vi "GetCutData.vi"(8 "error in (no error)":errorcluster, 9 "CustomMarking":T1={"CustomMarkVar"="JointAngles", "CustomMarkVarIdx"=0}, 10 "CutVar":T2, 11 "CAlexData":refnum<class "CAlex2_Data.lvclass">) -> (0 "error out":errorcluster, 1 "MarkingVar":dbl[](array[numeric]), 2 "Time":dbl[](array[numeric]), 3 "CAlexData out":refnum<class "CAlex2_Data.lvclass">, 4 "MarkingVar3":dbl[][](array[numeric]))   [LabVIEW 2016, in "CAlex2_Data.lvclass"]
uses:
  CAlex2_Data.lvclass
  cutvar.ctl
  D:/JinXin/LabVIEW.git/CAlex2-Controller-master/Sim&Process/DataProcess/ExpData/ExpData.lvclass
  CAlex2_Data.lvclass/CAlex2_Data.ctl
  Classes/CAlex2/CAlex2.lvclass
  D:/JinXin/LabVIEW.git/CAlex2-Controller-master/Classes/SerialChain-Cable/SerialChain-Cable.lvclass
  ExpData/ExpData.lvclass
  Classes/SerialChain-Cable/SerialChain-Cable.lvclass
panel:
  out "Waveform Graph":dbl[][](graph)
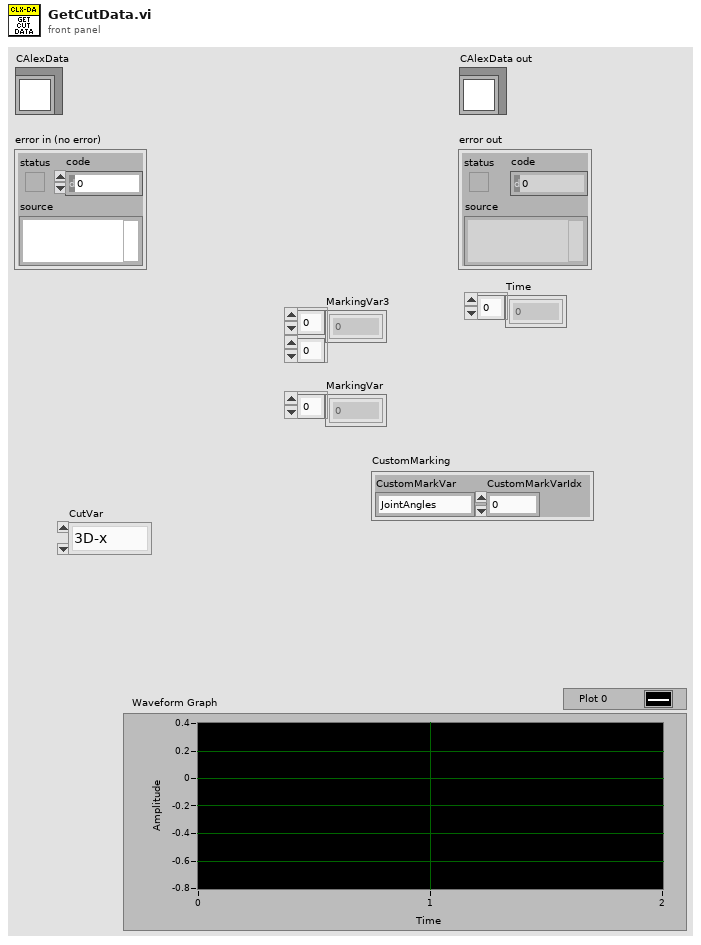
[diagram p1: front panel]
types:
  T1 = cluster{"CustomMarkVar":string, "CustomMarkVarIdx":i32}
  T2 = typedef "CAlex2_Data.lvclass/cutvar.ctl" = enum16{"3D-x", "2D-x", "Custom"}
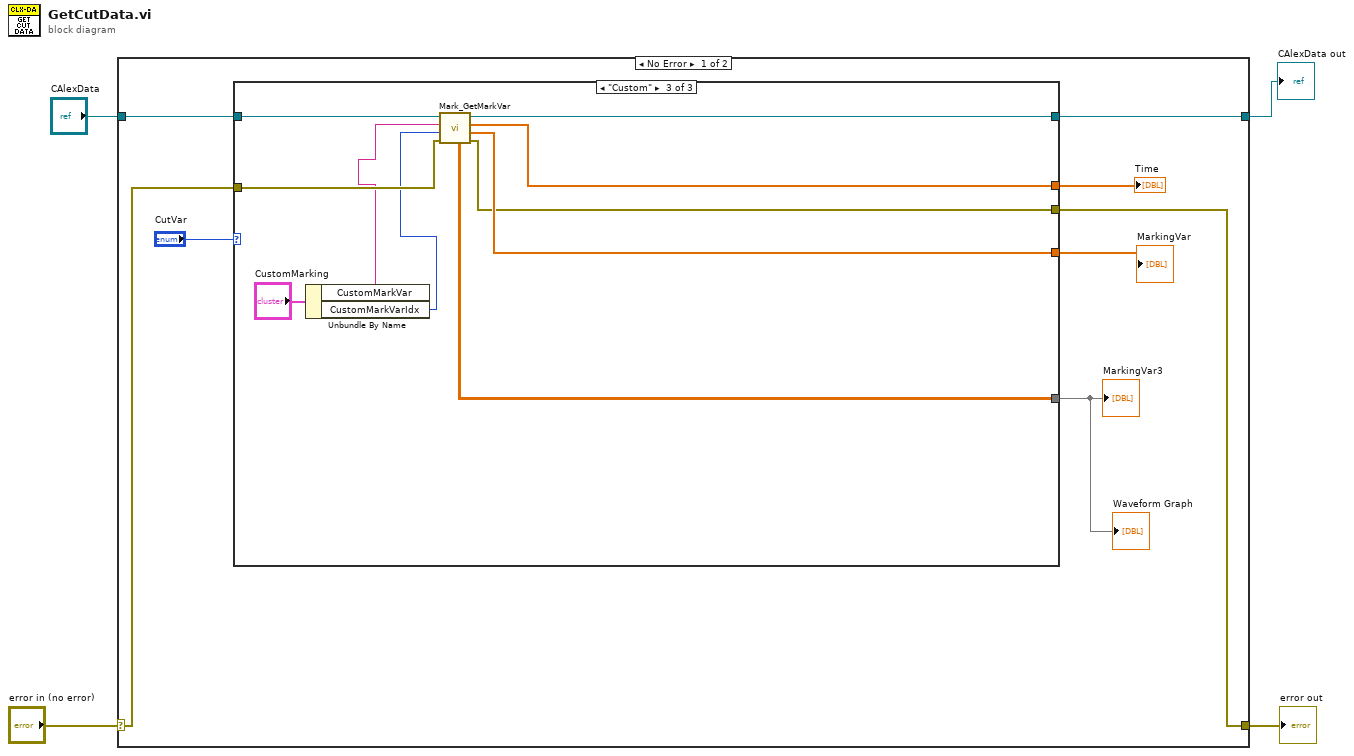
[diagram p0: block diagram]
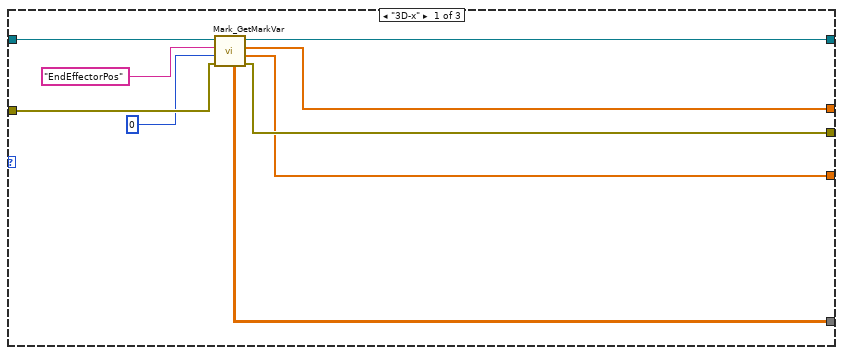
[diagram p2: hidden frame]
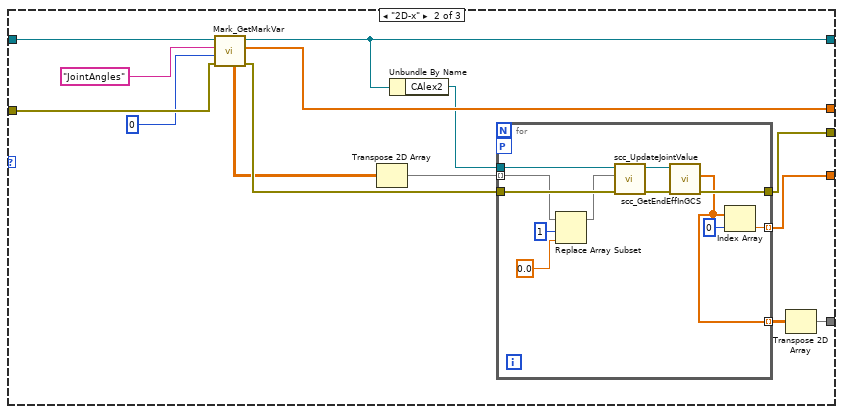
[diagram p3: hidden frame]
diagram:
  n1 = case shown="No Error" "error in (no error)" {
    selector: "error in (no error)" -> [w9 w59]
    tunnel: [w8 w59] -> w3
    tunnel: [w10 w58] -> w1
    tunnel: "CAlexData" -> [w11 w58]
    frame No Error {
      n2 = case shown="\"Custom\"" "CutVar" {
        tunnel: w11 -> [w21 w35 w57]
        tunnel: [w20 w30 w54] -> w10
        tunnel: [w19 w25 w51] -> w8
        tunnel: w9 -> [w18 w34 w56]
        tunnel: [w17 w26 w52] -> w6
        tunnel: [w14 w31 w55] -> w7
        tunnel: [w13 w22 w53] -> w5
        frame "3D-x" {
          n3 = call "Mark_GetMarkVar.vi"("error in (no error)"=w18, "VarIdx(0)"=0 ("MarkingVarIdx"), "VarName"="EndEffectorPos" ("MarkingVar"), "ExpData in"=w21) -> ("error out"=w19:errorcluster, "Var"=w17:dbl[], "Time"=w14:dbl[], "ExpData out"=w20:refnum<class "CAlex2_Data.lvclass">, "Var_All"=w13:dbl[][])  [unwired: 3 in]
        }
        frame "2D-x" {
          n4 = call "Mark_GetMarkVar.vi"("error in (no error)"=w34, "VarIdx(0)"=0 ("MarkingVarIdx"), "VarName"="JointAngles" ("MarkingVar"), "ExpData in"=w35) -> ("error out"=w29:errorcluster, "Time"=w31:dbl[], "ExpData out"=w30:refnum<class "CAlex2_Data.lvclass">, "Var_All"=w28:dbl[][])  [unwired: 3 in, 1 out]
          n5 = Transpose 2D Array(2D array=w28) -> (transposed array=w23:dbl[][])
          n6 = Unbundle By Name(w30) -> ("CAlex2"=w27:refnum<class "CAlex2.lvclass">)
          n7 = for {
            tunnel: w23 -> [w40] mode=indexing
            tunnel: [w41] -> w26 mode=indexing
            tunnel: [w36] -> w24 mode=indexing
            tunnel: w27 -> [w45]
            workers-P: _ -> [_]
            tunnel: w29 -> [w44]
            tunnel: [w43] -> w25
            n8 = Replace Array Subset(array=w40, new element=0.0 ("new element/subarray"), index=1) -> (w39:dbl[])
            n9 = call-dynamic "scc_UpdateJointValue.vi"("error in (no error)"=w44, "JointValue (rad|m)"=w39, "C-Alex in"=w45) -> ("error out"=w47:errorcluster, "C-Alex out"=w46:refnum<class "CAlex2.lvclass">)  [unwired: 7 in]
            n10 = call "scc_GetEndEffInGCS.vi"("error in (no error)"=w47, "SerialChain_Cable in"=w46) -> ("error out"=w43:errorcluster, "Pendeff(GCS)"=w36:dbl[])  [unwired: 5 in, 3 out]
            n11 = Index Array(array=w36, index=0) -> (element=w41:dbl)
          }
          n12 = Transpose 2D Array(2D array=w24) -> (transposed array=w22:dbl[][])
        }
        frame "Custom" {
          n13 = Unbundle By Name("CustomMarking") -> ("CustomMarkVar"=w49:string, "CustomMarkVarIdx"=w48:i32)
          n14 = call "Mark_GetMarkVar.vi"("error in (no error)"=w56, "VarIdx(0)"=w48, "VarName"=w49, "ExpData in"=w57) -> ("error out"=w51:errorcluster, "Var"=w52:dbl[], "Time"=w55:dbl[], "ExpData out"=w54:refnum<class "CAlex2_Data.lvclass">, "Var_All"=w53:dbl[][])  [unwired: 3 in]
        }
      }
      "Time" <- w7
      "MarkingVar3" <- w5
      "MarkingVar" <- w6
      "Waveform Graph" <- w5
    }
    frame Error {
    }
  }
  "error out" <- w3
  "CAlexData out" <- w1
